vi "Add Parameter Data.vi"(8 "error in (no error)":errorcluster, 10 "step parameters":T1, 11 "test step in":refnum<class "NI SystemLink Test Step.lvclass">) -> (0 "error out":errorcluster, 3 "test step out":refnum<class "NI SystemLink Test Step.lvclass">)   [LabVIEW 2018]
uses:
  <vilib>/Skyline/TestMonitor/Test Step/NI SystemLink Test Step.lvclass
  <vilib>/Skyline/Utilities/Property.ctl
  <vilib>/Skyline/TestMonitor/Test Step/Test Step Data.ctl
  <vilib>/Skyline/Utilities/NI Skyline Utilities.lvlib
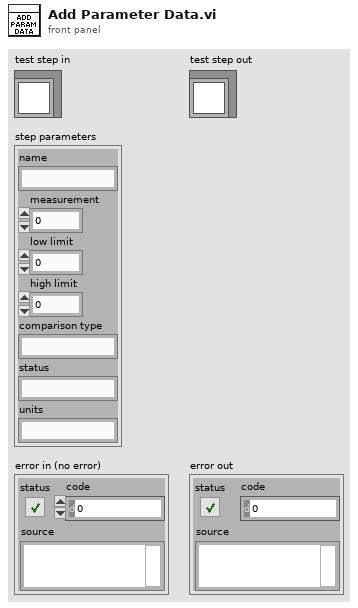
[diagram p1: front panel]
types:
  T1 = cluster{"name":string, "measurement":dbl, "low limit":dbl, "high limit":dbl, "comparison type":string, "status":string, "units":string}
  T2 = typedef "NI SystemLink Test Step.lvclass/Test Step Data.ctl" = cluster{"text":string, "parameters":cluster{"parameter list":T3[]}[]}
  T3 = typedef "NI Skyline Utilities.lvlib/Property.ctl" = cluster{"key":string, "value":string}
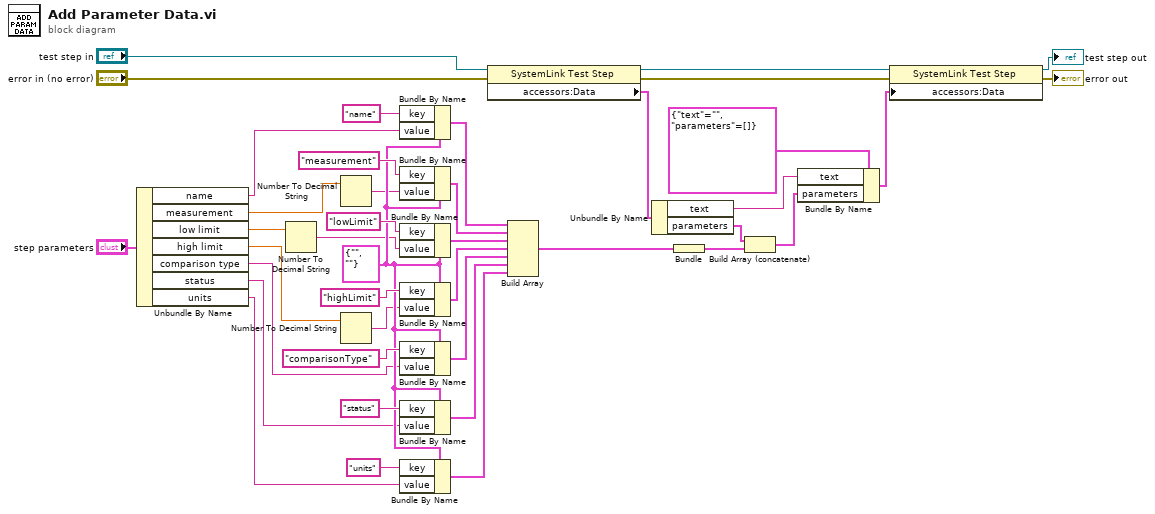
[diagram p0: block diagram]
diagram:
  w33 = T3 {"key"="", "value"=""} ("parameter")
  n1 = Unbundle By Name("step parameters") -> ("name"=w21:string, "measurement"=w16:dbl, "low limit"=w17:dbl, "high limit"=w18:dbl, "comparison type"=w19:string, "status"=w20:string, "units"=w15:string)
  n2 = Number To Decimal String(number=w17) -> (decimal integer string=w31:string)  [unwired: 1 in]
  n3 = Number To Decimal String(number=w16) -> (decimal integer string=w30:string)  [unwired: 1 in]
  n4 = Number To Decimal String(number=w18) -> (decimal integer string=w32:string)  [unwired: 1 in]
  n5 = Bundle By Name(cluster=w33, "key"="name", "value"=w21) -> (w29:T3)
  n6 = Bundle By Name(cluster=w33, "key"="measurement", "value"=w30) -> (w28:T3)
  n7 = Bundle By Name(cluster=w33, "key"="lowLimit", "value"=w31) -> (w27:T3)
  n8 = Bundle By Name(cluster=w33, "key"="highLimit", "value"=w32) -> (w26:T3)
  n9 = Bundle By Name(cluster=w33, "key"="comparisonType", "value"=w19) -> (w25:T3)
  n10 = Bundle By Name(cluster=w33, "key"="status", "value"=w20) -> (w24:T3)
  n11 = Bundle By Name(cluster=w33, "key"="units", "value"=w15) -> (w23:T3)
  n12 = property class="SystemLink Test Step"(reference="test step in", error in="error in (no error)") -> (reference out=w5:refnum<class "NI SystemLink Test Step.lvclass">, error out=w3:errorcluster, "accessors:Data"=w11:T2)
  n13 = Build Array(w29, w28, w27, w26, w25, w24, w23) -> (w22:T3[])
  n14 = Unbundle By Name(w11) -> ("text"=w7:string, "parameters"=w10:cluster{"parameter list":T3[]}[])
  n15 = Bundle(w22) -> (w9:cluster{T3[]})  [unwired: 1 in]
  n16 = Build Array (concatenate)(w10, w9) -> (w8:cluster{"parameter list":T3[]}[])
  n17 = Bundle By Name(cluster=T2 {"text"="", "parameters"=[]} ("Data"), "text"=w7, "parameters"=w8) -> (w6:T2)
  n18 = property class="SystemLink Test Step"(reference=w5, error in=w3, "accessors:Data"=w6) -> (reference out=→"test step out":refnum<class "NI SystemLink Test Step.lvclass">, error out=→"error out":errorcluster)
